vi "27-Host Requests to Enter On-Line.vi"(8 "error in (no error)":errorcluster, 11 "On-Line":bool) -> (0 "error out":errorcluster, 2 "Timeout?":bool, 3 "S1F18":T1)   [LabVIEW 2020, in "SECS Scenarios.lvlib" / "Scenarios Class.lvclass"]
uses:
  Scenarios Class.lvclass
  SECS Communication/S1 Message Class/S1F18.ctl
  27-Host Requests to Enter On-Line.ctl
  SECS Communication/S1 Message Class/S1 Message Class.lvclass
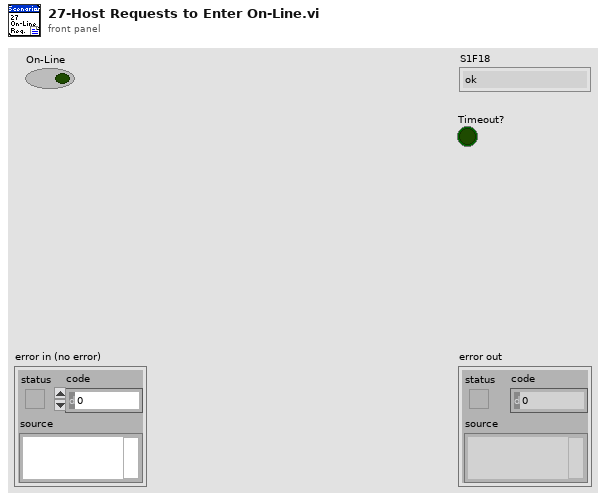
[diagram p1: front panel]
types:
  T1 = typedef "SECS Communication.lvlib/S1 Message Class.lvclass/S1F18.ctl" = enum16{"ok", "refused", "already online"}
  T2 = typedef "SECS Scenarios.lvlib/Scenarios Class.lvclass/27-Host Requests to Enter On-Line.ctl" = cluster{"On-Line":bool, "Reply Notifier":refnum<notifier>}
  T3 = typedef "SECS Scenarios.lvlib/Scenarios Class.lvclass/Broadcast Refnum.ctl" = cluster{"13-EnableDisable Alarm":refnum<user-event>, "15-Process Program Request":refnum<user-event>, "16-Process Program Send":refnum<user-event>, "17-Deleting a Process Program by Host":refnum<user-event>, "18-Host Requests Equipment Process Program Directory":refnum<user-event>, "19-Equipment Process Program Uploading":refnum<user-event>, "20[1]-Process Program Downloading":refnum<user-event>, "20[2]-Process Program Downloading":refnum<user-event>, "22-Host Sends Information to Equipment":refnum<user-event>, "26-Host Requests to Enter OFF-Line":refnum<user-event>, "27-Host Requests to Enter On-Line":refnum<user-event>, "28[1]-Remote Control[PP-SELECT]":refnum<user-event>, "28[2]-Remote Control[START]":refnum<user-event>, "28[3]-Remote Control[STOP]":refnum<user-event>, "28[4]-Remote Control[LOCAL]":refnum<user-event>, "28[5]-Remote Control[REMOTE]":refnum<user-event>, "28[6]-Remote Control[RCMD]":refnum<user-event>, "30-Host Requests Equipment to Set Time":refnum<user-event>, "31-Host Requests Time Value from Equipment":refnum<user-event>, "32[1]-Trace Data Collection":refnum<user-event>, "32[2]-Trace Data Collection":refnum<user-event>}
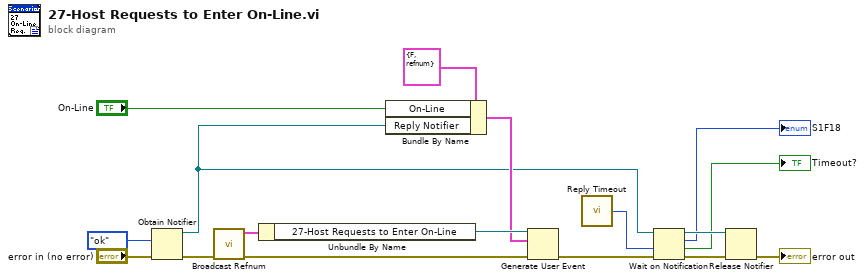
[diagram p0: block diagram]
diagram:
  n1 = Obtain Notifier(notification data type=S1F18."ok" ("S1F18"), error in (no error)="error in (no error)") -> (notifier out=w2:refnum<notifier>, error out=w16:errorcluster)  [unwired: 2 in, 1 out]
  n2 = call "Broadcast Refnum.vi"("error in"=w16) -> ("error out"=w15:errorcluster, "Broadcast Refnum"=w17:T3)  [unwired: 9 in]
  n3 = Unbundle By Name(w17) -> ("27-Host Requests to Enter On-Line"=w14:refnum<user-event>)
  n4 = Bundle By Name(cluster=T2 {"On-Line"=FALSE, "Reply Notifier"=refnum} ("27-Host Requests to Enter On-Line"), "On-Line"="On-Line", "Reply Notifier"=w2) -> (w5:T2)
  n5 = Generate User Event(user event=w14, event data cluster=w5, error in=w15) -> (error out=w13:errorcluster)  [unwired: 1 in, 1 out]
  n6 = call "Reply Timeout.vi"() -> ("Reply Timeout"=w12:i32)
  n7 = Wait on Notification(notifier=w2, timeout in ms (-1)=w12, error in (no error)=w13) -> (notifier out=w11:refnum<notifier>, notification=→"S1F18":T1, timed out?=→"Timeout?":bool, error out=w10:errorcluster)  [unwired: 1 in]
  n8 = Release Notifier(notifier=w11, error in (no error)=w10) -> (error out=→"error out":errorcluster)  [unwired: 1 in, 2 out]
